vi "Pre Launch Init.vi"(11 "MainActor in":refnum<class "MainActor.lvclass">) -> (0 "error out":errorcluster, 3 "MainActor out":refnum<class "MainActor.lvclass">)   [LabVIEW 2025, in "MainActor.lvlib" / "MainActor.lvclass"]
doc: "<p>(<strong>Filename</strong>: <span class=\"dnl\">Actor Framework.lvlib:Actor.lvclass:Pre Launch Init.vi</span>)</p>\n<p>Defines behavior that occurs after the <a href=\"nihelplauncher://docs/csh?context=lvcore_lvcomm_af_launch_nested_actor\">Launch Nested Actor</a> method is invoked but before the actor's Actor Core method begins running.</p>\n<p>By default, this method does nothing. A descendant class may override it to define behavior.</p>"
uses:
  MainActor.lvclass
  <vilib>/ActorFramework/Actor/Actor.lvclass
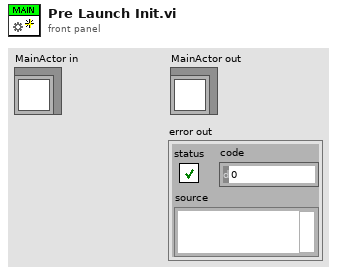
[diagram p1: front panel]
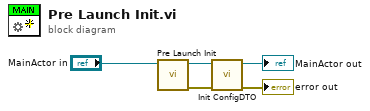
[diagram p0: block diagram]
diagram:
  n1 = call-parent "Pre Launch Init.vi"("Actor in"="MainActor in") -> ("error out"=w4:errorcluster, "Actor out"=w2:refnum<class "MainActor.lvclass">)  [unwired: 9 in]
  n2 = call "Init ConfigDTO.vi"("error in (no error)"=w4, "MainActor in"=w2) -> ("error out"=→"error out":errorcluster, "MainActor out"=→"MainActor out":refnum<class "MainActor.lvclass">)  [unwired: 8 in]
